vi "Splines.vi"(8 "Points":dbl[][](array[numeric])=[[-200.0, -0.1], [-400.0, -0.2], [-600.0, -0.5], [-800.0, -100.0]], 10 "P2i":T1, 11 "P1i":T1) -> (3 "Spline":cluster{dbl[], dbl[]})   [LabVIEW 2015]
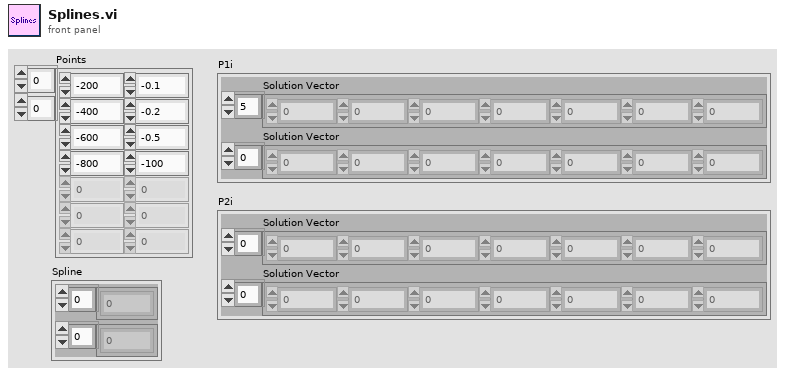
[diagram p1: front panel]
types:
  T1 = cluster{"Solution Vector":dbl[], "Solution Vector":dbl[]}
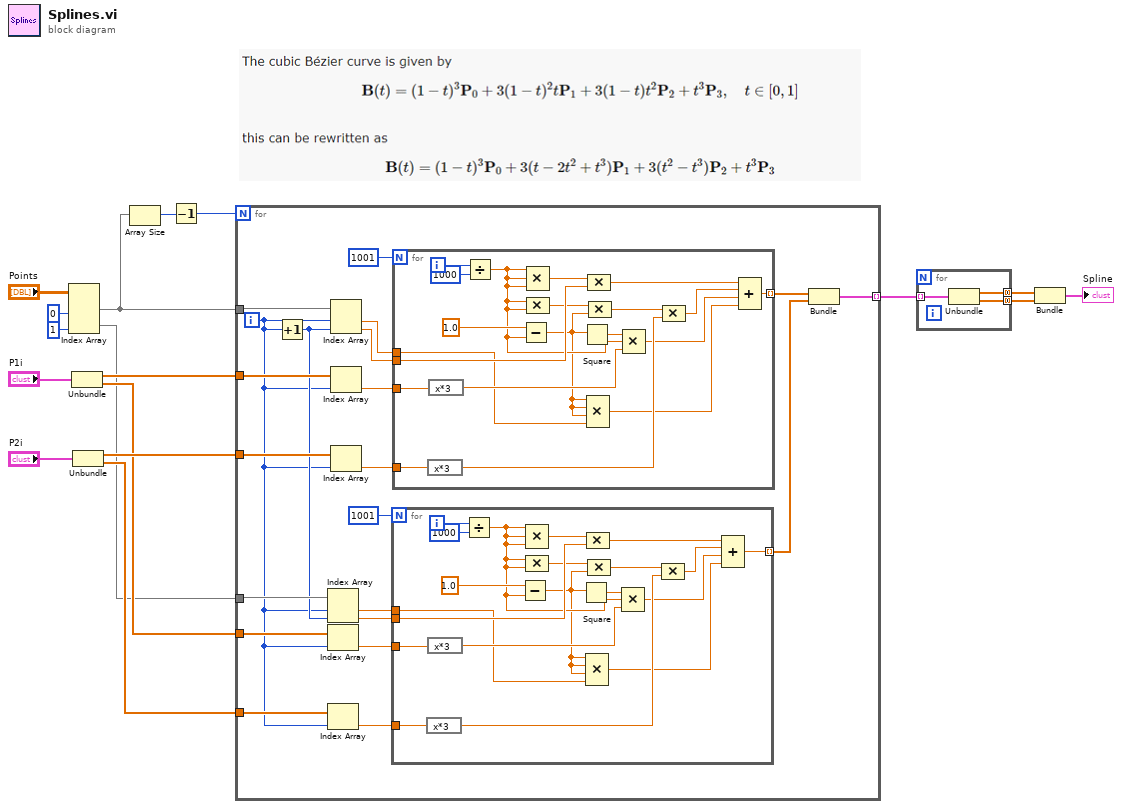
[diagram p0: block diagram]
diagram:
  n1 = Index Array(array="Points", index (col) #1=0 ("disabled index (col)"), index (col) #2=1 ("index (col)")) -> (element #1=w6:dbl[], element #2=w2:dbl[])  [unwired: 2 in]
  n2 = Unbundle("P1i") -> ("Solution Vector"=w13:dbl[], "Solution Vector"=w12:dbl[])
  n3 = Unbundle("P2i") -> ("Solution Vector"=w14:dbl[], "Solution Vector"=w11:dbl[])
  n4 = Array Size(array=w6) -> (size(s)=w5:i32)
  n5 = Decrement(x=w5) -> (x-1=w4:i32)
  n6 = for {
    N: w4 -> [_]
    tunnel: w6 -> [w37]
    tunnel: w14 -> [w36]
    tunnel: w13 -> [w35]
    tunnel: w12 -> [w25]
    tunnel: w11 -> [w24]
    tunnel: w2 -> [w29]
    tunnel: [w21] -> w3 mode=indexing
    i -> [w18]
    n7 = Increment(x=w18) -> (x+1=w26:i32)
    n8 = Index Array(array=w29, index #1=w18, index #2=w26) -> (element #1=w28:dbl, element #2=w27:dbl)
    n9 = Index Array(array=w25, index=w18) -> (element=w23:dbl)
    n10 = Index Array(array=w24, index=w18) -> (element=w22:dbl)
    n11 = Index Array(array=w37, index #1=w18, index #2=w26) -> (element #1=w34:dbl, element #2=w33:dbl)
    n12 = Index Array(array=w35, index=w18) -> (element=w32:dbl)
    n13 = Index Array(array=w36, index=w18) -> (element=w31:dbl)
    n14 = for {
      N: 1001 -> [_]
      tunnel: w27 -> [w55]
      tunnel: w23 -> [w54]
      tunnel: w22 -> [w53]
      tunnel: w28 -> [w40]
      tunnel: [w39] -> w19 mode=indexing
      i -> [w41]
      n15 = expression code="x*3"(w53) -> (w48:dbl)
      n16 = expression code="x*3"(w54) -> (w47:dbl)
      n17 = Divide(x=w41, y=1000) -> (x/y=w50:dbl)
      n18 = Subtract(x=1.0, y=w50) -> (x-y=w43:dbl)
      n19 = Compound Arithmetic op=MULTIPLY(w50, w50, w50) -> (w56:dbl)
      n20 = Compound Arithmetic op=MULTIPLY(w50, w50) -> (w52:dbl)
      n21 = Square(x=w43) -> (x^2=w51:dbl)
      n22 = Compound Arithmetic op=MULTIPLY(w43, w43, w43, w40) -> (w42:dbl)
      n23 = Compound Arithmetic op=MULTIPLY(w56, w55) -> (w46:dbl)
      n24 = Compound Arithmetic op=MULTIPLY(w52, w43) -> (w49:dbl)
      n25 = Compound Arithmetic op=MULTIPLY(w51, w50, w47) -> (w44:dbl)
      n26 = Compound Arithmetic op=MULTIPLY(w49, w48) -> (w45:dbl)
      n27 = Compound Arithmetic op=ADD(w46, w45, w44, w42) -> (w39:dbl)
    }
    n28 = for {
      N: 1001 -> [_]
      tunnel: w33 -> [w74]
      tunnel: w32 -> [w73]
      tunnel: w31 -> [w72]
      tunnel: [w62] -> w20 mode=indexing
      tunnel: w34 -> [w59]
      i -> [w78]
      n29 = expression code="x*3"(w72) -> (w67:dbl)
      n30 = expression code="x*3"(w73) -> (w66:dbl)
      n31 = Divide(x=w78, y=1000) -> (x/y=w69:dbl)
      n32 = Subtract(x=1.0, y=w69) -> (x-y=w61:dbl)
      n33 = Compound Arithmetic op=MULTIPLY(w69, w69, w69) -> (w75:dbl)
      n34 = Compound Arithmetic op=MULTIPLY(w69, w69) -> (w71:dbl)
      n35 = Square(x=w61) -> (x^2=w70:dbl)
      n36 = Compound Arithmetic op=MULTIPLY(w61, w61, w61, w59) -> (w60:dbl)
      n37 = Compound Arithmetic op=MULTIPLY(w75, w74) -> (w65:dbl)
      n38 = Compound Arithmetic op=MULTIPLY(w71, w61) -> (w68:dbl)
      n39 = Compound Arithmetic op=MULTIPLY(w70, w69, w66) -> (w63:dbl)
      n40 = Compound Arithmetic op=MULTIPLY(w68, w67) -> (w64:dbl)
      n41 = Compound Arithmetic op=ADD(w65, w64, w63, w60) -> (w62:dbl)
    }
    n42 = Bundle(w20, w19) -> (w21:cluster{dbl[], dbl[]})  [unwired: 1 in]
  }
  n43 = for {
    tunnel: w3 -> [w81] mode=indexing
    tunnel: [w80] -> w10 mode=concatenating
    tunnel: [w79] -> w1 mode=concatenating
    n44 = Unbundle(w81) -> (w80:dbl[], w79:dbl[])
  }
  n45 = Bundle(w10, w1) -> (→"Spline":cluster{dbl[], dbl[]})  [unwired: 1 in]
